vi "Init.vi"(6 "Priority (F)":bool, 8 "error in (no error)":errorcluster, 11 "Data":variant) -> (0 "error out":errorcluster)   [LabVIEW 2020, in "UI.lvlib"]
uses:
  UI.lvlib
  Private Controls/Element.ctl
  Private Controls/Module Action.ctl
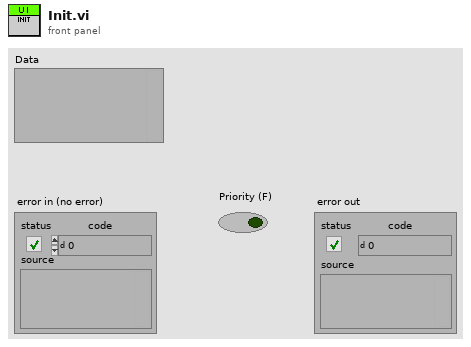
[diagram p1: front panel]
types:
  T1 = typedef "UI.lvlib/Module Action.ctl" = enum16{"Initialise Module", "Connect", "Setup", "Pause", "Start", "Search", "Set IP", "Count Call", "Update Progress Bar", "Update UI", "Stop", "Post Results", "Wait: Time Elapsed", "Error", "Exit"}
  T2 = typedef "UI.lvlib/Element.ctl" = cluster{"Action":T1, "Data":variant}
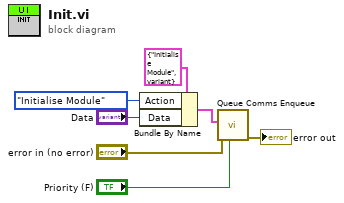
[diagram p0: block diagram]
diagram:
  n1 = Bundle By Name(cluster=T2 {"Action"=enum."Initialise Module", "Data"=variant} ("Element"), "Action"=Module_Action."Initialise Module", "Data"="Data") -> (w1:T2)
  n2 = call "Queue Comms Enqueue.vi"("Priority (F)"="Priority (F)", "error in (no error)"="error in (no error)", "Element"=w1) -> ("error out"=→"error out":errorcluster)  [unwired: 8 in]
